vi "GVSMove Docking Graph.vi"(9 "StartPositin In":T1, 10 "MousePositin In":T1, 11 "VI Ref In":refnum<vi>) -> (0 "bResult":bool, 1 "StartPositin Out":T1, 3 "VI Ref Out":refnum<vi>)   [LabVIEW 2013]
uses:
  <vilib>/Utility/miscctls.llb/LVRectTypeDef.ctl
  GVSNew View Global.vi
panel:
  out "Start_Positin 2":T1
  in  "ToolBar Click":bool
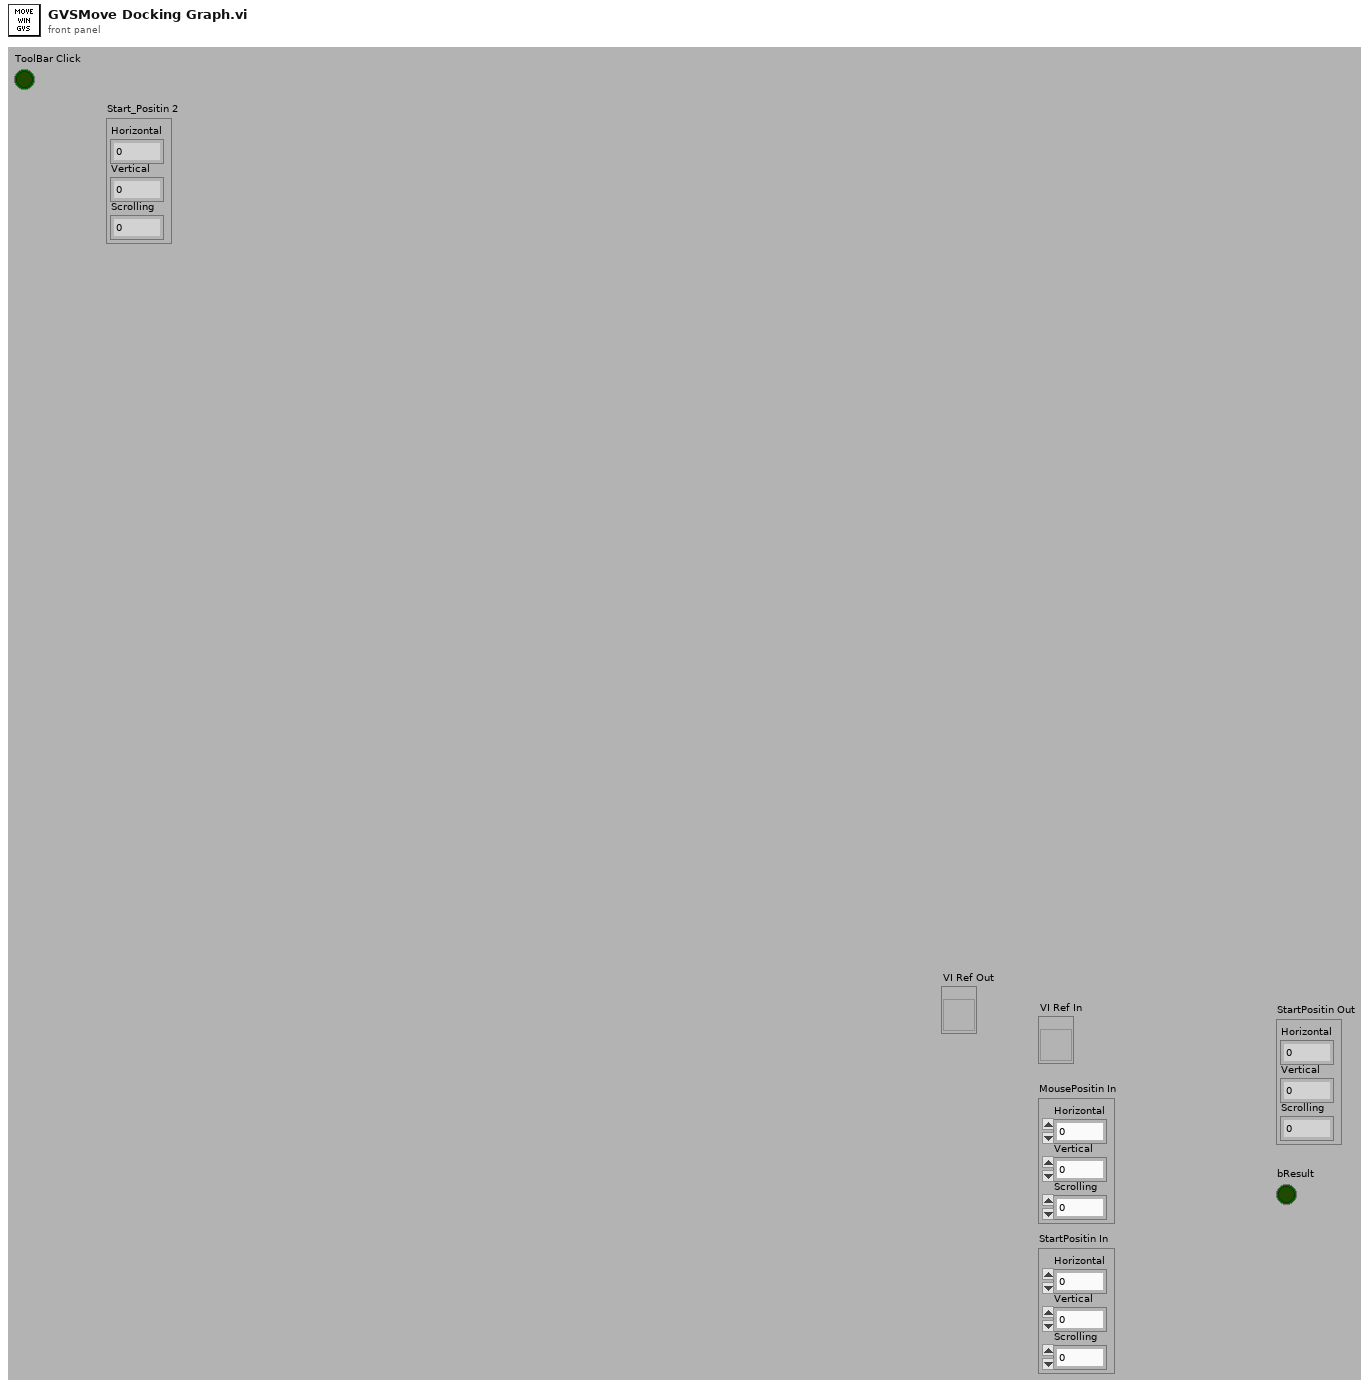
[diagram p1: front panel]
types:
  T1 = cluster{"Horizontal":i32, "Vertical":i32, "Scrolling":i32}
  T2 = typedef "LVRectTypeDef.ctl" = cluster{"Left":i16, "Top":i16, "Right":i16, "Bottom":i16}
  T3 = enum32{"Invalid", "Standard", "Closed", "Hidden", "Minimized", "Maximized"}
  T4 = cluster{"Horizontal":bool, "Vertical":bool, "Scrolling":bool}
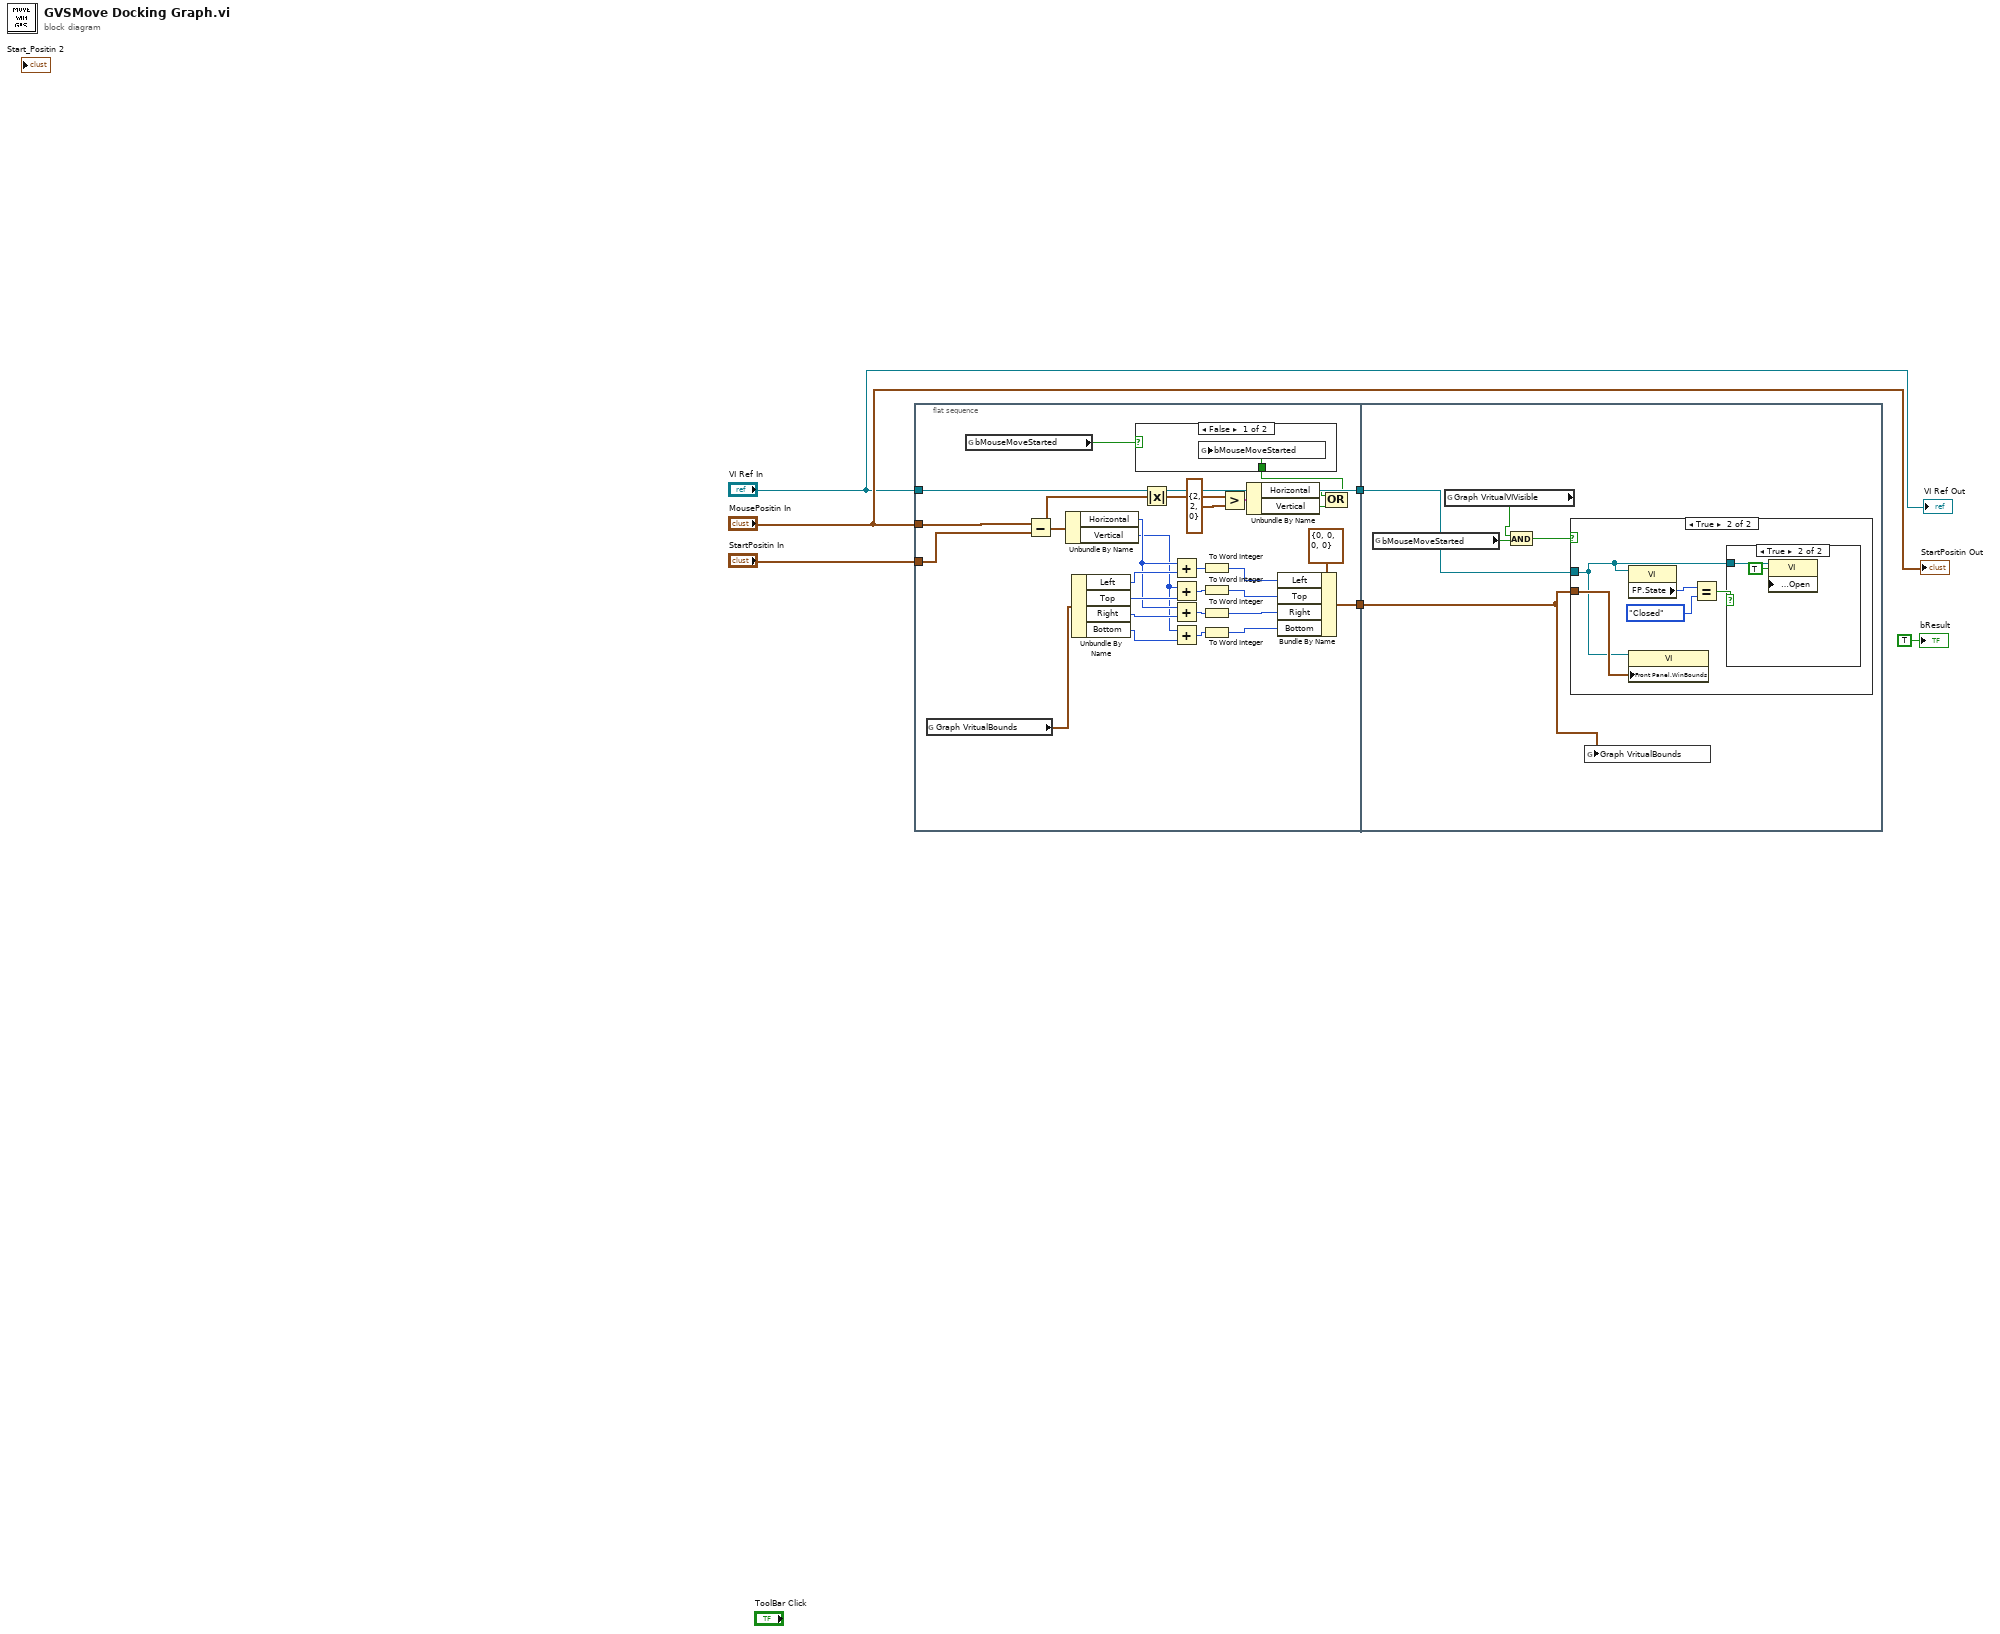
[diagram p0: block diagram]
diagram:
  n1 = flat-sequence {
    tunnel: "MousePositin In" -> [w24]
    tunnel: "StartPositin In" -> [w23]
    tunnel: [w17] -> w6
    tunnel: [w16] -> w5
    tunnel: "VI Ref In" -> [w16]
    tunnel: w6 -> [w39]
    tunnel: w5 -> [w40]
    frame #0 {
      n2 = global read "GVSNew View Global.vi" "Graph VritualBounds"() -> (w15:T2)
      n3 = global read "GVSNew View Global.vi" "bMouseMoveStarted"() -> (w8:bool)
      n4 = Subtract(x=w24, y=w23) -> (x-y=w10:T1)
      n5 = Unbundle By Name(w10) -> ("Horizontal"=w30:i32, "Vertical"=w29:i32)
      n6 = Unbundle By Name(w15) -> ("Left"=w34:i16, "Top"=w33:i16, "Right"=w32:i16, "Bottom"=w31:i16)
      n7 = Absolute Value(x=w10) -> (abs(x)=w9:T1)
      n8 = Add(x=w30, y=w34) -> (x+y=w28:i32)
      n9 = Add(x=w29, y=w33) -> (x+y=w27:i32)
      n10 = Add(x=w30, y=w32) -> (x+y=w26:i32)
      n11 = Add(x=w29, y=w31) -> (x+y=w25:i32)
      n12 = To Word Integer(number=w28) -> (16bit integer=w18:i16)
      n13 = To Word Integer(number=w27) -> (16bit integer=w19:i16)
      n14 = To Word Integer(number=w26) -> (16bit integer=w20:i16)
      n15 = To Word Integer(number=w25) -> (16bit integer=w21:i16)
      n16 = Greater?(x=w9, y=T1 {"Horizontal"=2, "Vertical"=2, "Scrolling"=0}) -> (0:w13:T4)
      n17 = Unbundle By Name(w13) -> ("Horizontal"=w12:bool, "Vertical"=w11:bool)
      n18 = Bundle By Name(cluster=T2 {"Left"=0, "Top"=0, "Right"=0, "Bottom"=0} ("Front Panel Window:Window Bounds"), "Left"=w18, "Top"=w19, "Right"=w20, "Bottom"=w21) -> (w17:T2)
      n19 = Compound Arithmetic op=OR(w12, w11) -> (w7:bool)
      n20 = case shown="False" w8 {
        tunnel: w7 -> [w35 _]
        frame False {
          n21 = global write "GVSNew View Global.vi" "bMouseMoveStarted"(w35) -> ()
        }
        frame True {
        }
      }
    }
    frame #1 {
      n22 = global read "GVSNew View Global.vi" "bMouseMoveStarted"() -> (w36:bool)
      n23 = global read "GVSNew View Global.vi" "Graph VritualVIVisible"() -> (w37:bool)
      n24 = And(x=w37, y=w36) -> (x .and. y?=w38:bool)
      n25 = case shown="True" w38 {
        tunnel: w40 -> [_ w44]
        tunnel: w39 -> [_ w45]
        frame False {
        }
        frame True {
          n26 = property class="VI"(reference=w44) -> ("FP.State"=w43:T3)  [unwired: 1 in, 2 out]
          n27 = property class="VI"(reference=w44, "Front Panel.WinBounds"=w45) -> ()  [unwired: 1 in, 2 out]
          n28 = Equal?(x=w43, y=T3."Closed" ("Front Panel Window:State")) -> (x = y?=w41:bool)
          n29 = case shown="True" w41 {
            tunnel: w44 -> [_ w46]
            frame False {
            }
            frame True {
              n30 = property class="VI"(reference=w46, "Front Panel.Open"=TRUE ("Front Panel Window:Open")) -> ()  [unwired: 1 in, 2 out]
            }
          }
        }
      }
      n31 = global write "GVSNew View Global.vi" "Graph VritualBounds"(w39) -> ()
    }
  }
  "StartPositin Out" <- "MousePositin In"
  "bResult" <- TRUE ("bResult")
  "VI Ref Out" <- "VI Ref In"
